vi "Handle Event.vi"(8 "error in (no error)":errorcluster, 9 "Event Data":refnum<class "Event.lvclass">, 11 "Controller in":refnum<class "Controller.lvclass">) -> (0 "error out":errorcluster, 3 "Controller out":refnum<class "Controller.lvclass">)   [LabVIEW 2023, in "MVC Actors.lvlib" / "Controller.lvclass"]
uses:
  Controller.lvclass
  Event/Event.lvclass
  Controller.lvclass/Controller.ctl
  Event Handlers/Abstract Event Handler for Controller/Abstract Event Handler for Controller.lvclass
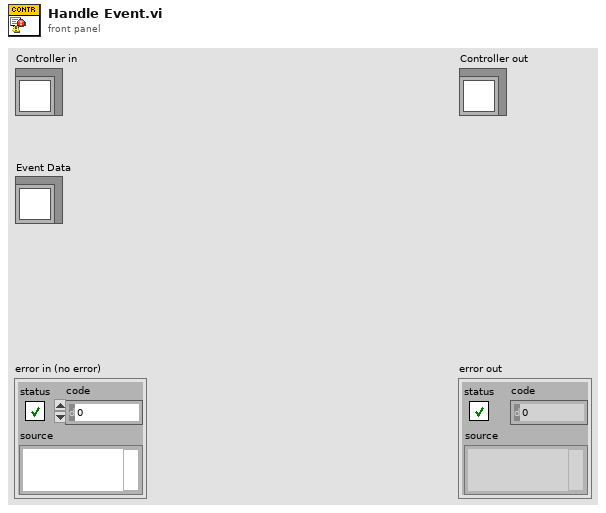
[diagram p1: front panel]
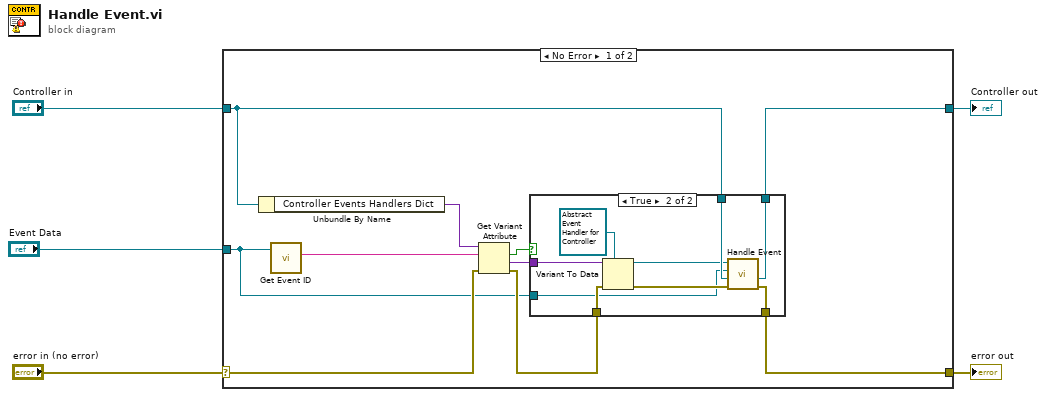
[diagram p0: block diagram]
diagram:
  n1 = case shown="No Error" "error in (no error)" {
    selector: "error in (no error)" -> [w11 w28]
    tunnel: [w6 w28] -> w4
    tunnel: [w8 w27] -> w1
    tunnel: "Controller in" -> [w7 w27]
    tunnel: "Event Data" -> [w9 _]
    frame No Error {
      n2 = Unbundle By Name(w7) -> ("Controller Events Handlers Dict"=w15:variant)
      n3 = call-dynamic "Get Event ID.vi"("Event in"=w9) -> ("Event ID"=w14:string)  [unwired: 8 in, 2 out]
      n4 = Get Variant Attribute(Variant=w15, name=w14, error in=w11) -> (found=w13:bool, value=w12:variant, error out=w10:errorcluster)  [unwired: 1 in, 1 out]
      n5 = case shown="True" w13 {
        tunnel: w12 -> [_ w26]
        tunnel: w10 -> [w17 w24]
        tunnel: w7 -> [w16 w20]
        tunnel: [w16 w23] -> w8
        tunnel: [w17 w22] -> w6
        tunnel: w9 -> [_ w19]
        frame False {
        }
        frame True {
          n6 = Variant To Data(error in=w24, type=refnum<class "Abstract Event Handler for Controller.lvclass"> refnum ("Source Event Fire Handler"), Variant=w26) -> (data=w18:refnum<class "Abstract Event Handler for Controller.lvclass">, error out=w21:errorcluster)
          n7 = call-dynamic "Handle Event.vi"("error in (no error)"=w21, "Controller in"=w20, "Event Data"=w19, "Abstract Event Handler for Controller in"=w18) -> ("error out"=w22:errorcluster, "Controller out"=w23:refnum<class "Controller.lvclass">)  [unwired: 5 in, 1 out]
        }
      }
    }
    frame Error {
    }
  }
  "error out" <- w4
  "Controller out" <- w1
